vi "HovaCAL Setpoints.vi"(7 "running":bool, 11 "TestKonfig (Eingang)":T1 {"TestKonfig Interferent"."Gasflasche MFC3" items=["----"=10000, "IAG NH3 3000"=0, "IAG NH3 200"=1, "IAG NH3 2000"=2, "IAG MG"=3, "IAG O2"=4]; "TestKonfig Interferent"."Gasflasche MFC2" items=["----"=10000, "IAG NH3 3000"=0, "IAG NH3 200"=1, "IAG NH3 2000"=2, "IAG MG"=3, "IAG O2"=4]; "TestKonfig Interferent"."Eingangs Konzentration MFC1" min=0.0; "TestKonfig Interferent"."Ausgangs Konzentration MFC1" min=0.0; "TestKonfig Interferent"."MFC2" items=["MFC 2", "MFC 3", "MFC 4", "MFC 5"]; "TestKonfig Interferent"."MFC3" items=["MFC 2", "MFC 3", "MFC 4", "MFC 5"]; "TestKonfig Interferent"."Ausgangs Konzentration MFC3" min=0.0; "TestKonfig Interferent"."Eingangs Konzentration MFC3" min=0.0; "TestKonfig Interferent"."Ausgangs Konzentration MFC2" min=0.0; "TestKonfig Interferent"."Eingangs Konzentration MFC2" min=0.0; "TestKonfig H2O"."HovaCAL Temperature" format="%.2f"; "TestKonfig H2O"."HovaCAL Flow Input Cluster"."HovaCAL Flow Input Cluster" format="%.2f"; "TestKonfig H2O"."Eingangs Konzentration:" min=0.0; "TestKonfig H2O"."zusätzliche Zeitdauer Erster Punkt" min=30 step=1 format="%#_5g"; "TestKonfig H2O"."Zeitdauer Stufen" format="%#_5g"; "TestKonfig H2O"."Max Fehler" format="%#_5g"; "TestKonfig H2O"."Anzahl Stufen" format="%#_5g"; "TestKonfig H2O"."Modus" items=["Messen", "CG zu Entnahmestelle"]}) -> (3 "TestKonfig (Ausgang)":T1 {"TestKonfig Interferent"."Gasflasche MFC3" items=["----"=10000, "IAG NH3 3000"=0, "IAG NH3 200"=1, "IAG NH3 2000"=2, "IAG MG"=3, "IAG O2"=4]; "TestKonfig Interferent"."Gasflasche MFC2" items=["----"=10000, "IAG NH3 3000"=0, "IAG NH3 200"=1, "IAG NH3 2000"=2, "IAG MG"=3, "IAG O2"=4]; "TestKonfig Interferent"."Eingangs Konzentration MFC1" min=0.0; "TestKonfig Interferent"."Ausgangs Konzentration MFC1" min=0.0; "TestKonfig Interferent"."MFC2" items=["MFC 2", "MFC 3", "MFC 4", "MFC 5"]; "TestKonfig Interferent"."MFC3" items=["MFC 2", "MFC 3", "MFC 4", "MFC 5"]; "TestKonfig Interferent"."Ausgangs Konzentration MFC3" min=0.0; "TestKonfig Interferent"."Eingangs Konzentration MFC3" min=0.0; "TestKonfig Interferent"."Ausgangs Konzentration MFC2" min=0.0; "TestKonfig Interferent"."Eingangs Konzentration MFC2" min=0.0; "TestKonfig H2O"."HovaCAL Temperature" format="%.2f"; "TestKonfig H2O"."HovaCAL Flow Input Cluster"."HovaCAL Flow Input Cluster" format="%.2f"; "TestKonfig H2O"."Eingangs Konzentration:" min=0.0; "TestKonfig H2O"."zusätzliche Zeitdauer Erster Punkt" min=30 step=1 format="%#_5g"; "TestKonfig H2O"."Zeitdauer Stufen" format="%#_5g"; "TestKonfig H2O"."Max Fehler" format="%#_5g"; "TestKonfig H2O"."Anzahl Stufen" format="%#_5g"; "TestKonfig H2O"."Modus" items=["Messen", "CG zu Entnahmestelle"]})   [LabVIEW 2020, in "EPA 1065.lvlib" / "HovaCAL Interference verificaton.lvlib"]
uses:
  HovaCAL Interference verificaton.lvlib
  TestKonfig.ctl
  TestKonfig H2O.ctl
  Modus.ctl
  Linearisierung V2/SpanEinstellungen/Einheit.ctl
  Linearisierung V2/Gasteiler/Stufen Tabelle 10 Stufen.ctl
  Linearisierung V2/Gasteiler/HovaCAL_Interface/Controls/Flow Einstellung.ctl
  Linearisierung V2/Gasteiler/HovaCAL_Interface/Controls/Temp Sollwerte Anzeige.ctl
  TestKonfig Interferents.ctl
  MFCAuswahl.ctl
  Seiten/System Einstellungen V2/Gasflasche Auswahl.ctl
  Linearisierung V2/Gasteiler/HovaCAL_Interface/Kommunikation/Kommunikation.lvlib
  Linearisierung V2/Gasteiler/HovaCAL_Interface/Kommunikation/Aktion_FGV_HovaCAL_Interface_SetData.ctl
  Linearisierung V2/SpanEinstellungen/SpanEinstellungen.lvlib
  Linearisierung V2/Gasteiler/HovaCAL_Interface/Controls/Controls.lvlib
  Seiten/System Einstellungen V2/System Einstellungen V2.lvlib
  Linearisierung V2/Gasteiler/Gasteiler.lvlib
panel:
  # "sec"
  # "%"
  # "sec"
  # "sec"
  # "%"
  # "sec"
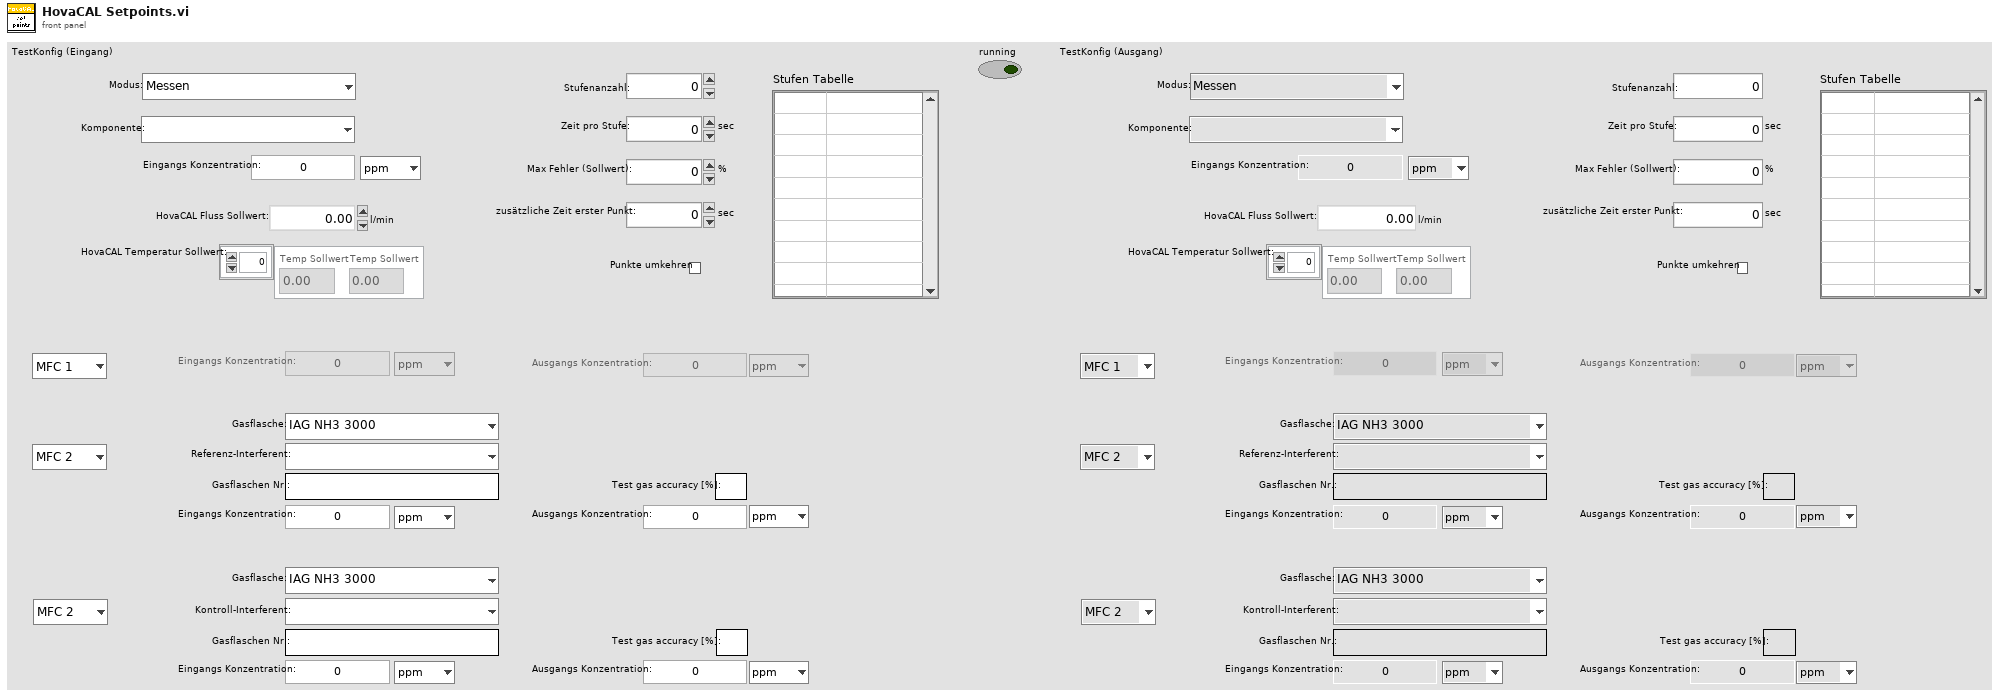
[diagram p1: front panel]
types:
  T1 = typedef "EPA 1065.lvlib/HovaCAL Interference verificaton.lvlib/TestKonfig.ctl" = cluster{"TestKonfig H2O":T2, "TestKonfig Interferent":T8}
  T2 = typedef "EPA 1065.lvlib/HovaCAL Interference verificaton.lvlib/TestKonfig H2O.ctl" = cluster{"Modus":T3, "Komponente:":u16, "Eingangs Konzentration:":dbl, "Einheit":T4, "Anzahl Stufen":sgl, "Zeitdauer Stufen":sgl, "Max Fehler":sgl, "zusätzliche Zeitdauer Erster Punkt":sgl, "Punkte umkehren":bool, "Stufen Tabelle":T5, "HovaCAL Flow Input Cluster":T6, "HovaCAL Temperature":T7}
  T3 = typedef "EPA 1065.lvlib/HovaCAL Interference verificaton.lvlib/Modus.ctl" = u16
  T4 = typedef "Linearisierung v2.lvlib/SpanEinstellungen.lvlib/Einheit.ctl" = enum16{"ppm", "%"}
  T5 = typedef "Linearisierung v2.lvlib/Gasteiler.lvlib/Stufen Tabelle 10 Stufen.ctl" = string[][]
  T6 = typedef "Linearisierung v2.lvlib/Gasteiler.lvlib/HovaCAL_Interface.lvlib/Controls.lvlib/Flow Einstellung.ctl" = cluster{"HovaCAL Flow Input Cluster":dbl}
  T7 = typedef "Linearisierung v2.lvlib/Gasteiler.lvlib/HovaCAL_Interface.lvlib/Controls.lvlib/Temp Sollwerte Anzeige.ctl" = dbl[]
  T8 = typedef "EPA 1065.lvlib/HovaCAL Interference verificaton.lvlib/TestKonfig Interferents.ctl" = cluster{"MFC1":enum16{"MFC 1"}, "Eingangs Konzentration MFC1":dbl, "Einheit MFC1 Eingang":T4, "Ausgangs Konzentration MFC1":dbl, "Einheit MFC1 Ausgang":T4, "MFC2":T9, "Referenz-Interferent:":u16, "Gasflaschen Nr MFC2":string, "Accuracy MFC2":string, "Eingangs Konzentration MFC2":dbl, "Einheit MFC2 Eingang":T4, "Ausgangs Konzentration MFC2":dbl, "Einheit MFC2 Ausgang":T4, "MFC3":T9, "Kontroll-Interferent:":u16, "Gasflaschen Nr MFC3":string, "Accuracy MFC3":string, "Eingangs Konzentration MFC3":dbl, "Einheit MFC3 Eingang":T4, "Ausgangs Konzentration MFC3":dbl, "Einheit MFC3 Ausgang":T4, "Gasflasche MFC2":T10, "Gasflasche MFC3":T10}
  T9 = typedef "EPA 1065.lvlib/HovaCAL Interference verificaton.lvlib/MFCAuswahl.ctl" = u16
  T10 = typedef "System Einstellungen V2.lvlib/Gasflasche Auswahl.ctl" = u16
  T11 = typedef "Linearisierung v2.lvlib/Gasteiler.lvlib/HovaCAL_Interface.lvlib/Kommunikation.lvlib/Aktion_FGV_HovaCAL_Interface_SetData.ctl" = enum16{"lesen", "Konzentrationen", "Pumpen Parameter", "Pumpe Konzentration", "Pumpe run", "Temperaturen", "Fluss", "Limits", "init"}
  T12 = cluster{"input concentration setpoint":dbl, "output concentration setpoint":dbl}[]
  T13 = cluster{"input concentration setpoint":dbl, "output concentration setpoint":dbl}
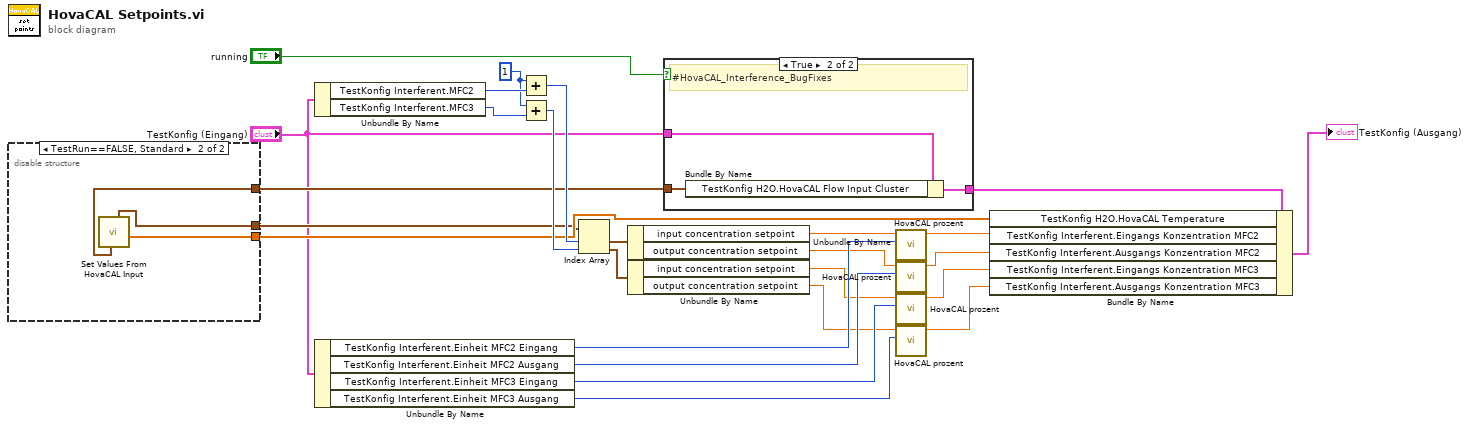
[diagram p0: block diagram]
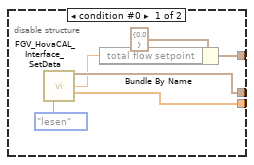
[diagram p3: hidden frame]
diagram:
  w23 = u16 1 ("x+y")
  n1 = disable-structure shown="TestRun==FALSE, Standard" {
    disable-tunnel: [w30 w35] -> w6
    disable-tunnel: [w31 w34] -> w5
    disable-tunnel: [w28 w33] -> w4
    frame condition #0 {
      n2 = call "FGV_HovaCAL_Interface_SetData.vi"("Aktion"=Aktion_FGV_HovaCAL_Interface_SetData."lesen") -> ("Set Values Cluster out"=w31:T12, "total flow setpoint out"=w27:dbl, "Temperature out"=w30:dbl[])  [unwired: 8 in, 4 out]
      n3 = Bundle By Name(cluster=cluster{"total flow setpoint":dbl} {"total flow setpoint"=0.0} ("Flow Input Cluster"), "total flow setpoint"=w27) -> (w28:cluster{"total flow setpoint":dbl})
    }
    frame condition #1 (active) {
      n4 = call "Set Values From HovaCAL Input.vi"() -> ("HovaCAL Temperature"=w35:dbl[], "Set Values Cluster"=w34:T12, "Flow Input Cluster"=w33:cluster{"total flow setpoint":dbl})  [unwired: 3 in, 6 out]
    }
  }
  n5 = Unbundle By Name("TestKonfig (Eingang)") -> ("TestKonfig Interferent.MFC2"=w25:T9, "TestKonfig Interferent.MFC3"=w24:T9)
  n6 = Unbundle By Name("TestKonfig (Eingang)") -> ("TestKonfig Interferent.Einheit MFC2 Eingang"=w17:T4, "TestKonfig Interferent.Einheit MFC2 Ausgang"=w14:T4, "TestKonfig Interferent.Einheit MFC3 Eingang"=w11:T4, "TestKonfig Interferent.Einheit MFC3 Ausgang"=w8:T4)
  n7 = Add(x=w23, y=w25) -> (x+y=w22:T9)
  n8 = Add(x=w23, y=w24) -> (x+y=w21:T9)
  n9 = Index Array(array=w5, index #1=w22, index #2=w21) -> (element #1=w20:T13, element #2=w19:T13)
  n10 = Unbundle By Name(w20) -> ("input concentration setpoint"=w18:dbl, "output concentration setpoint"=w15:dbl)
  n11 = Unbundle By Name(w19) -> ("input concentration setpoint"=w12:dbl, "output concentration setpoint"=w9:dbl)
  n12 = case shown="True" "running" {
    tunnel: w4 -> [_ w39]
    tunnel: "TestKonfig (Eingang)" -> [w36 w38]
    tunnel: [w36 w37] -> w2
    frame False {
    }
    frame True {
      # "#HovaCAL_Interference_BugFixes"
      n13 = Bundle By Name(cluster=w38, "TestKonfig H2O.HovaCAL Flow Input Cluster"=w39) -> (w37:T1)
    }
  }
  n14 = call "HovaCAL prozent.vi"("Einheit MFC2 Eingang"=w17, "Eingangs Konzentration MFC2"=w18) -> ("Numerisch"=w16:dbl)  [unwired: 9 in]
  n15 = call "HovaCAL prozent.vi"("Einheit MFC2 Eingang"=w14, "Eingangs Konzentration MFC2"=w15) -> ("Numerisch"=w13:dbl)  [unwired: 9 in]
  n16 = call "HovaCAL prozent.vi"("Einheit MFC2 Eingang"=w11, "Eingangs Konzentration MFC2"=w12) -> ("Numerisch"=w10:dbl)  [unwired: 9 in]
  n17 = call "HovaCAL prozent.vi"("Einheit MFC2 Eingang"=w8, "Eingangs Konzentration MFC2"=w9) -> ("Numerisch"=w7:dbl)  [unwired: 9 in]
  n18 = Bundle By Name(cluster=w2, "TestKonfig H2O.HovaCAL Temperature"=w6, "TestKonfig Interferent.Eingangs Konzentration MFC2"=w16, "TestKonfig Interferent.Ausgangs Konzentration MFC2"=w13, "TestKonfig Interferent.Eingangs Konzentration MFC3"=w10, "TestKonfig Interferent.Ausgangs Konzentration MFC3"=w7) -> (→"TestKonfig (Ausgang)":T1)
